vi "Initialize Input Gain.vi"(8 "error in (no error)":errorcluster, 11 "Instrument.DAQ":refnum<class "Instrument.DAQ.lvclass">) -> (0 "error out":errorcluster, 2 "Input Gain":T1, 3 "Instrument.DAQ out":refnum<class "Instrument.DAQ.lvclass">)   [LabVIEW 2019, in "Instrument.Lockin.lvlib" / "Instrument.DAQ.lvclass"]
uses:
  Instrument.DAQ.lvclass
  Typedefs/Channel.Gain--Cluster--Array.ctl
  Typedefs/Channel.Gain--Cluster.ctl
  Instrument.DAQ.lvclass/Instrument.DAQ.ctl
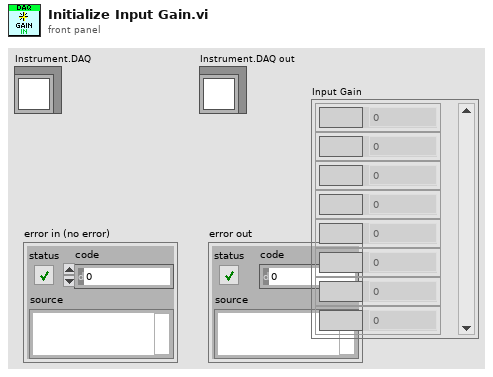
[diagram p1: front panel]
types:
  T1 = typedef "Instrument.Lockin.lvlib/Instrument.DAQ.lvclass/Channel.Gain--Cluster--Array.ctl" = T2[]
  T2 = typedef "Instrument.Lockin.lvlib/Instrument.DAQ.lvclass/Channel.Gain--Cluster.ctl" = cluster{"Channel":string, "Gain":dbl}
  T3 = typedef "Instrument.Lockin.lvlib/Instrument.DAQ.lvclass/DAQ.Config.AI--Cluster--Array.ctl" = T4[]
  T4 = typedef "Instrument.Lockin.lvlib/Instrument.DAQ.lvclass/DAQ.Config.AI--Cluster.ctl" = cluster{"Channels":tag, "Coupling":T5, "Range":T6, "input terminal configuration":i32, "Type":T7}
  T5 = typedef "Instrument.Lockin.lvlib/Instrument.DAQ.lvclass/DAQ.Config.AI.Coupling--enum.ctl" = u16
  T6 = typedef "Instrument.Lockin.lvlib/Instrument.DAQ.lvclass/DAQ.Config.AI.Range--enum.ctl" = enum16{"±0.316", "±1.00", "±3.16", "±10.0", "±31.6", "±42.4"}
  T7 = typedef "Instrument.Lockin.lvlib/Instrument.DAQ.lvclass/DAQ.Type--enum.ctl" = enum16{"None", "USB-4431", "PXI-446x"}
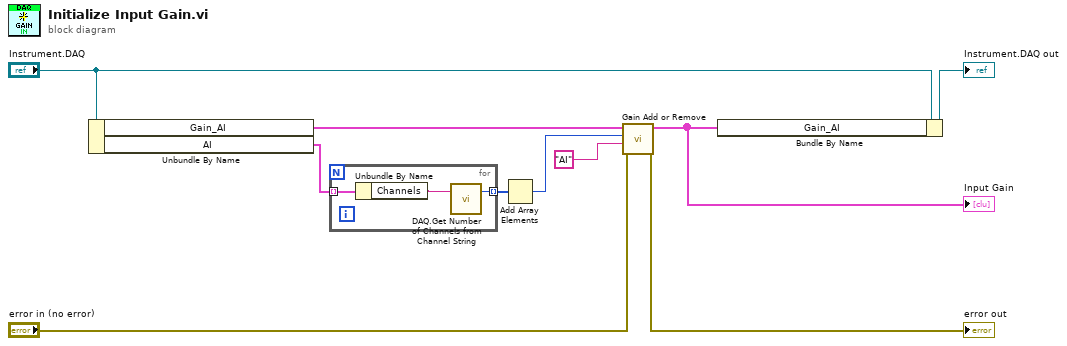
[diagram p0: block diagram]
diagram:
  n1 = Unbundle By Name("Instrument.DAQ") -> ("Gain_AI"=w7:T1, "AI"=w5:T3)
  n2 = for {
    tunnel: w5 -> [w13] mode=indexing
    tunnel: [w11] -> w10 mode=indexing
    n3 = Unbundle By Name(w13) -> ("Channels"=w12:tag)
    n4 = call "DAQ.Get Number of Channels from Channel String.vi"("Channels String"=w12) -> ("# channels"=w11:i32)  [unwired: 2 in]
  }
  n5 = Add Array Elements(numeric array=w10) -> (sum=w6:i32)
  n6 = call "Gain Add or Remove.vi"("error in (no error)"="error in (no error)", "Name Prefix"="AI", "Size"=w6, "Channel Gain"=w7) -> ("error out"=→"error out":errorcluster, "Channel Gain out"=w1:T1)  [unwired: 6 in]
  "Input Gain" <- w1
  n7 = Bundle By Name(cluster="Instrument.DAQ", "Gain_AI"=w1) -> (→"Instrument.DAQ out":refnum<class "Instrument.DAQ.lvclass">)
